vi "frequency measurement (array).vi"() -> (2 "real part of fft array":dbl[](array[numeric]))   [LabVIEW 2016]
uses:
  <vilib>/myRIO/Instrument Drivers/Onboard IO/AudioIn Block/typedefs/AudioIn Block Reference.ctl
  <vilib>/myRIO/Common/Instrument Driver Framework/Utilities/typedefs/myRIO Generic Hardware Reference.ctl
  <vilib>/myRIO/Common/Instrument Driver Framework/Utilities/typedefs/Hardware Version Enum.ctl
  <vilib>/myRIO/Common/Instrument Driver Framework/Utilities/typedefs/myRIO v1.0 Reference.ctl
  <vilib>/myRIO/Common/Instrument Driver Framework/Utilities/typedefs/Generic FPGA Reference.ctl
  <vilib>/myRIO/Common/Instrument Driver Framework/myRIO v1.0/AudioIn Block/typedefs/AudioIn Block Channels List.ctl
  <vilib>/myRIO/Common/Instrument Driver Framework/myRIO v1.0/AudioIn Block/typedefs/AudioIn Block Channels Enum.ctl
  <vilib>/myRIO/Common/Instrument Driver Framework/Utilities/typedefs/Analog Scaling Constants.ctl
  <vilib>/userdefined/High Color/nirio_resource_hc.ctl
  <vilib>/myRIO/Common/Instrument Driver Framework/Utilities/vis/Is FPGA Ref Available.vi
  <vilib>/myRIO/Common/Instrument Driver Framework/myRIO v1.0/AudioIn Block/vis/myRIO v1.1 Open Throughput AudioIn (N Samples).vi
  <vilib>/myRIO/Instrument Drivers/Onboard IO/AudioIn Block/vis/Read.vi
  <vilib>/Analysis/2dsp.llb/Real FFT.vi
  <vilib>/myRIO/Common/Instrument Driver Framework/Utilities/vis/Validate Channels.vi
  <vilib>/Utility/VariantDataType/GetNumericInfo.vi
  <vilib>/Utility/error.llb/Error Cluster From Error Code.vi
  <vilib>/myRIO/Common/Instrument Driver Framework/myRIO v1.0/myRIO v1.1 Open Throughput.vi
  <vilib>/myRIO/Common/Instrument Driver Framework/myRIO v1.0/AudioIn Block/vis/myRIO v1.0 Get Scaling Constants AudioIn Block.vi
  <vilib>/myRIO/Common/Instrument Driver Framework/myRIO v1.0/AudioIn Block/vis/myRIO v1.0 Reserve AudioIn Block.vi
  <vilib>/myRIO/Common/Instrument Driver Framework/myRIO v1.0/myRIO v1.0 Close.vi
  <vilib>/myRIO/Common/Instrument Driver Framework/myRIO v1.0/AudioIn Block/vis/myRIO v1.0 AudioIn Block Read.vi
  <vilib>/myRIO/Express VI/Onboard IO/AudioIn/AudioIn Express VI.xnode
  <vilib>/myRIO/Instrument Drivers/Onboard IO/AudioIn Block/vis/myRIO AudioIn N Samples Open.xnode
  <vilib>/myRIO/Instrument Drivers/Onboard IO/AudioIn Block/AudioIn Block.lvlib
  <vilib>/Analysis/NI_AALPro.lvlib
panel:
  out "Before":dbl[](graph)
  # "Size of the array is 1000, the frequency is equal to the array index * 2"
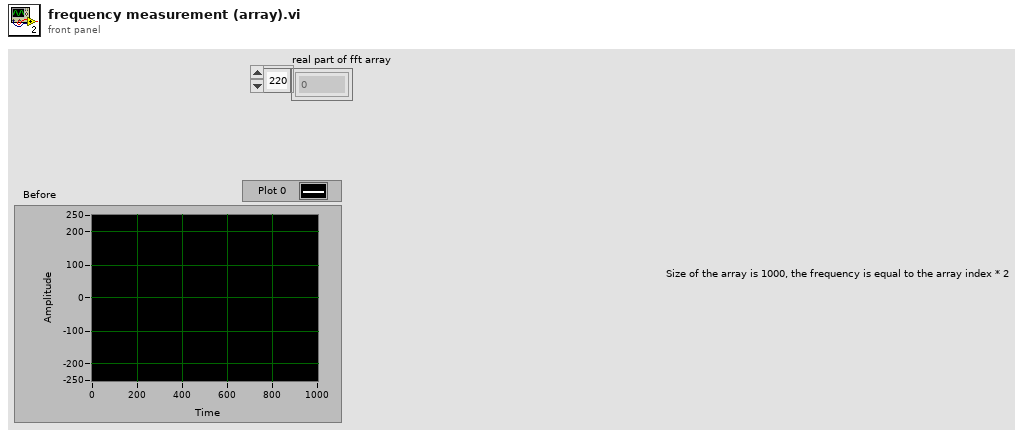
[diagram p1: front panel]
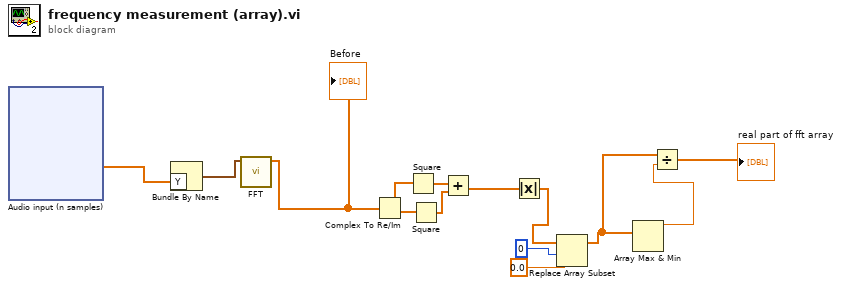
[diagram p0: block diagram]
diagram:
  n1 = xnode "Audio input (n samples)"() -> ("AudioIn/Left (N Samples)"=w14:dbl[])  [unwired: 1 in, 2 out]
  n2 = Bundle By Name("Y"=w14) -> (w13:waveform(dbl))  [unwired: 1 in]
  n3 = call-poly <vilib>:"FFT.vi"("X"=w13) -> ("FFT {X}"=w12:cdb[])  [unwired: 9 in, 1 out]
  "Before" <- w12
  n4 = Complex To Re/Im(x + iy=w12) -> (x=w10:dbl[], y=w11:dbl[])
  n5 = Square(x=w10) -> (x^2=w9:dbl[])
  n6 = Square(x=w11) -> (x^2=w8:dbl[])
  n7 = Add(x=w9, y=w8) -> (x+y=w7:dbl[])
  n8 = Absolute Value(x=w7) -> (abs(x)=w4:dbl[])
  n9 = Replace Array Subset(array=w4, new element=0.0 ("new element/subarray"), index=0) -> (w3:dbl[])
  n10 = Array Max & Min(array=w3) -> (max value=w2:dbl)  [unwired: 3 out]
  n11 = Divide(x=w3, y=w2) -> (x/y=→"real part of fft array":dbl[])
